vi "plc_start_stop_fgv.vi"(7 "Enum":T1, 8 "error in (no error)":errorcluster, 10 "Boolean":bool) -> (0 "error out":errorcluster, 2 "Boolean 2":bool)   [LabVIEW 2017]
uses:
  Control/FGV_Start_Stop.ctl
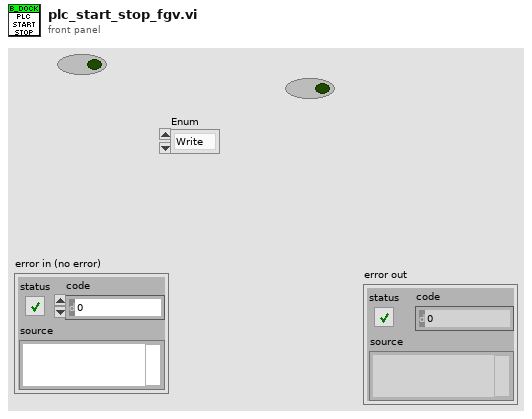
[diagram p1: front panel]
types:
  T1 = typedef "FGV_Start_Stop.ctl" = enum16{"Write", "Read"}
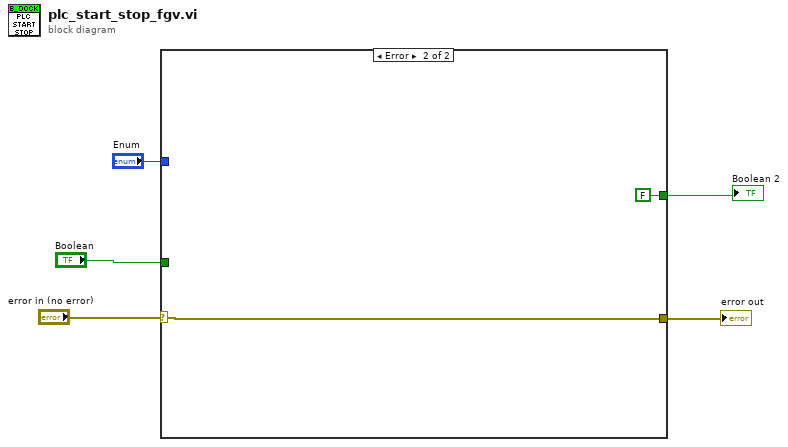
[diagram p0: block diagram]
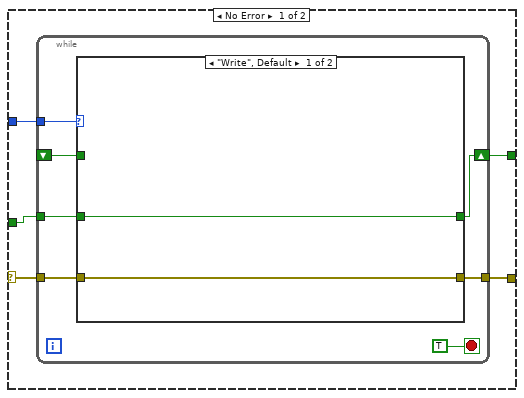
[diagram p2: hidden frame]
diagram:
  n1 = case shown="Error" "error in (no error)" {
    selector: "error in (no error)" -> [w8 w23]
    tunnel: [w7 w23] -> w4
    tunnel: "Enum" -> [w10 _]
    tunnel: "Boolean" -> [w9 _]
    tunnel: [w6 FALSE ("Boolean")] -> w1
    frame No Error {
      n2 = while {
        shift-right: [w15] -> w6
        shift-left: _ -> [w13]
        tunnel: w10 -> [w16]
        tunnel: w9 -> [w14]
        tunnel: w8 -> [w12]
        tunnel: [w11] -> w7
        stop <- TRUE stop-if-true
        n3 = case shown="\"Write\", Default" w16 {
          tunnel: [w19 w21] -> w15
          tunnel: w14 -> [w19 _]
          tunnel: w13 -> [_ w21]
          tunnel: w12 -> [w18 w20]
          tunnel: [w18 w20] -> w11
          frame "Write", Default {
          }
          frame "Read" {
          }
        }
      }
    }
    frame Error {
    }
  }
  "error out" <- w4
  "Boolean 2" <- w1
